vi "AVI Video Initialise (Ref video).vi"(8 "error in (no error)":errorcluster, 11 "Timelapse folder path":path) -> (0 "error out":errorcluster)   [LabVIEW 2020]
uses:
  Typedefs/Channel Selector.ctl
  Global Variables/General Globals.vi
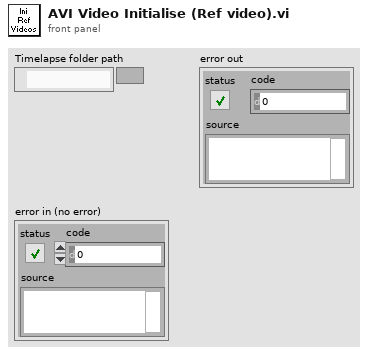
[diagram p1: front panel]
types:
  T1 = typedef "Channel Selector.ctl" = enum16{"Red Channel", "Green Channel", "Blended"}
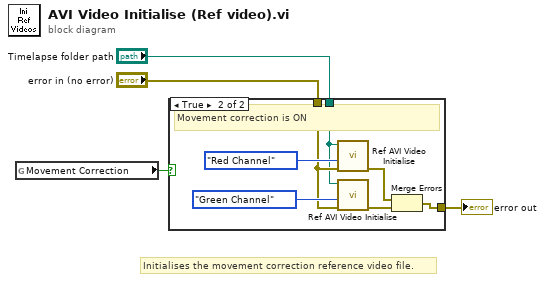
[diagram p0: block diagram]
diagram:
  # "Initialises the movement correction reference video file."
  n1 = global read "General Globals.vi" "Movement Correction"() -> (w4:bool)
  n2 = case shown="True" w4 {
    tunnel: "error in (no error)" -> [_ w9]
    tunnel: "Timelapse folder path" -> [_ w8]
    tunnel: [_ w5] -> w3
    frame False {
      # "Movement correction is OFF"
    }
    frame True {
      # "Movement correction is ON"
      n3 = call "Ref AVI Video Initialise.vi"("error in (no error)"=w9, "Channel"=Channel_Selector."Red Channel", "Timelapse folder path"=w8) -> ("error out"=w7:errorcluster)  [unwired: 8 in]
      n4 = call "Ref AVI Video Initialise.vi"("error in (no error)"=w9, "Channel"=Channel_Selector."Green Channel", "Timelapse folder path"=w8) -> ("error out"=w6:errorcluster)  [unwired: 8 in]
      n5 = Merge Errors(w7, w6) -> (w5:errorcluster)
    }
  }
  "error out" <- w3
